vi "Get STG wrapper.vi"(8 "error in (no error)":errorcluster caption="错误输入（无错误）", 9 "pStgInfo":T1, 10 "dwCanNodeId":u32, 11 "dwDevIndex":u32) -> (0 "error out":errorcluster caption="错误输出", 1 "pStgInfo out":T1, 3 "function return":u32)   [LabVIEW 2016, in "UISimCanFunc_wrapper.lvlib"]
doc: "_declspec (dllexport) DWORD GetSTG_wrapper(DWORD dwDevIndex, DWORD dwCanNodeId, P_STG_INFO_OBJ pStgInfo);"
uses:
  <userlib>/UISimCanFunc_wrapper/UISimCanFunc_wrapper.lvlib
  <userlib>/UISimCanFunc_wrapper/UISimCanFunc_wrapper.dll
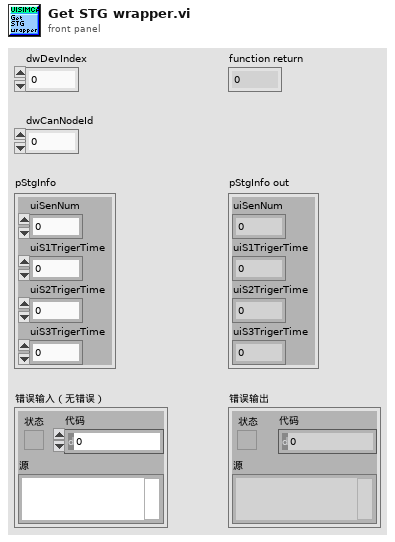
[diagram p1: front panel]
types:
  T1 = cluster{"uiSenNum":u32, "uiS1TrigerTime":u32, "uiS2TrigerTime":u32, "uiS3TrigerTime":u32}
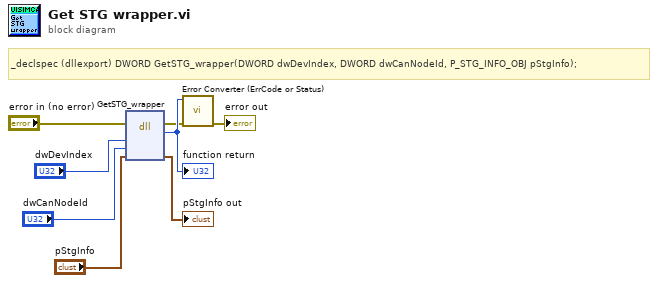
[diagram p0: block diagram]
diagram:
  # "_declspec (dllexport) DWORD GetSTG_wrapper(DWORD dwDevIndex, DWORD dwCanNodeId, P_STG_INFO_OBJ pStgInfo);"
  n1 = dll-call lib="C:/Program Files (x86)/National Instruments/LabVIEW 2016/user.lib/UISimCanFunc_wrapper/UISimCanFunc_wrapper.*" fn="GetSTG_wrapper"(error in="error in (no error)", "dwDevIndex"="dwDevIndex", "dwCanNodeId"="dwCanNodeId", "pStgInfo"="pStgInfo") -> (error out=w2:errorcluster, w8:u32, "pStgInfo"=→"pStgInfo out":T1)  [unwired: 4 in, 1 out]
  "function return" <- w8
  n2 = call <userlib>:"Error Converter (ErrCode or Status).vi"("error in (no error)"=w2, "error code"=w8) -> ("error out"=→"error out":errorcluster)  [unwired: 9 in]
